vi "Graph InitScale(XY).vi"(8 "error in (no error)":errorcluster caption="エラー入力（エラーなし）", 9 "XYグラフ(Nプロット)":cluster{"X配列":dbl[], "Y配列":dbl[]}[](array[cluster]), 10 "ChName(XY)":string[](array[string]), 11 "XYグラフ(ref)":refnum<vi>) -> (0 "error out":errorcluster caption="エラー出力", 2 "OK":bool)   [LabVIEW 2014]
panel:
  in  "SAVE":bool
  in  "LOAD":bool
  in  "停止":bool
  in  "Y軸データ":T1(array[cluster])
  in  "プロットデータ":T2(array[cluster]) {"MAX" format="%#_6f"; "MIN" format="%#_6f"; "Y軸" items=["回転数", "A2", "A3", "A44", "A5", "A6", "A7", "A8"]}
  # "最大値"
  # "最小値"
  # "Y軸"
  # "表示範囲外！"
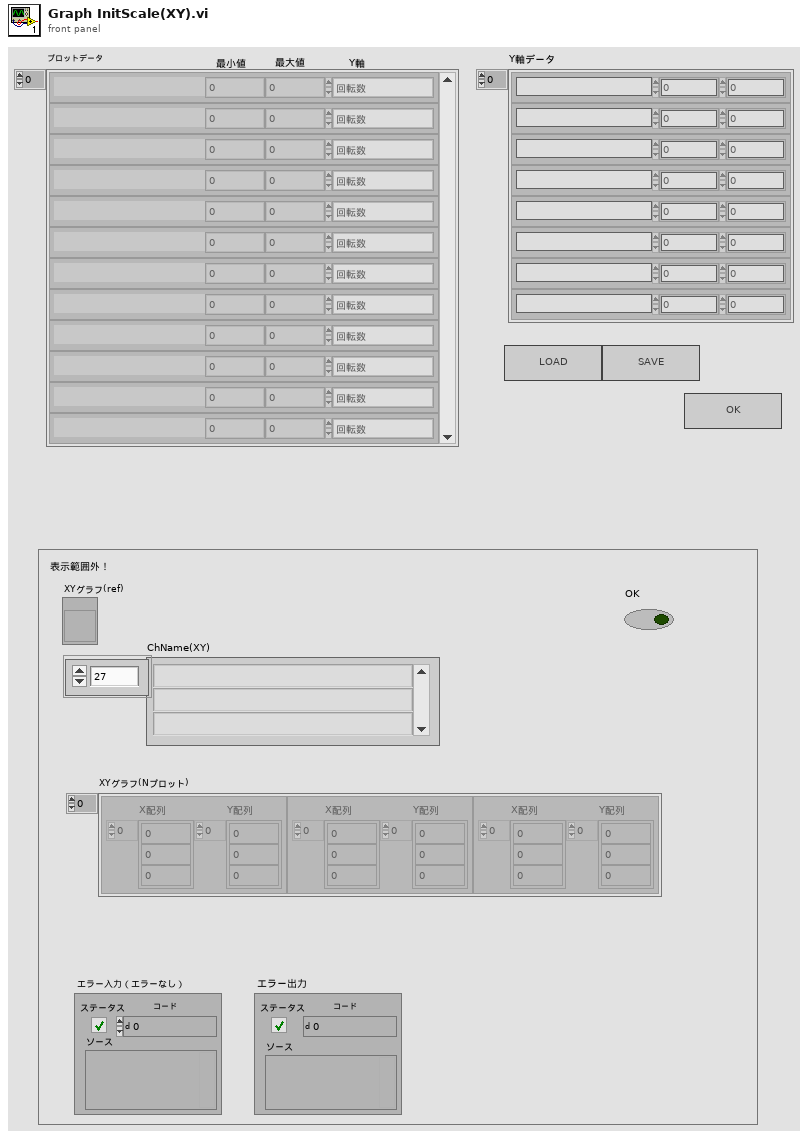
[diagram p1: front panel]
types:
  T1 = cluster{"YLegName":string, "MIN":dbl, "MAX":dbl}[]
  T2 = cluster{"CH名称":string, "MIN":dbl, "MAX":dbl, "Y軸":u16}[]
  T3 = enum32{"Invalid", "Standard", "Closed", "Hidden", "Minimized", "Maximized"}
  T4 = cluster{"CH名称":string, "MIN":dbl, "MAX":dbl, "Y軸":u16}
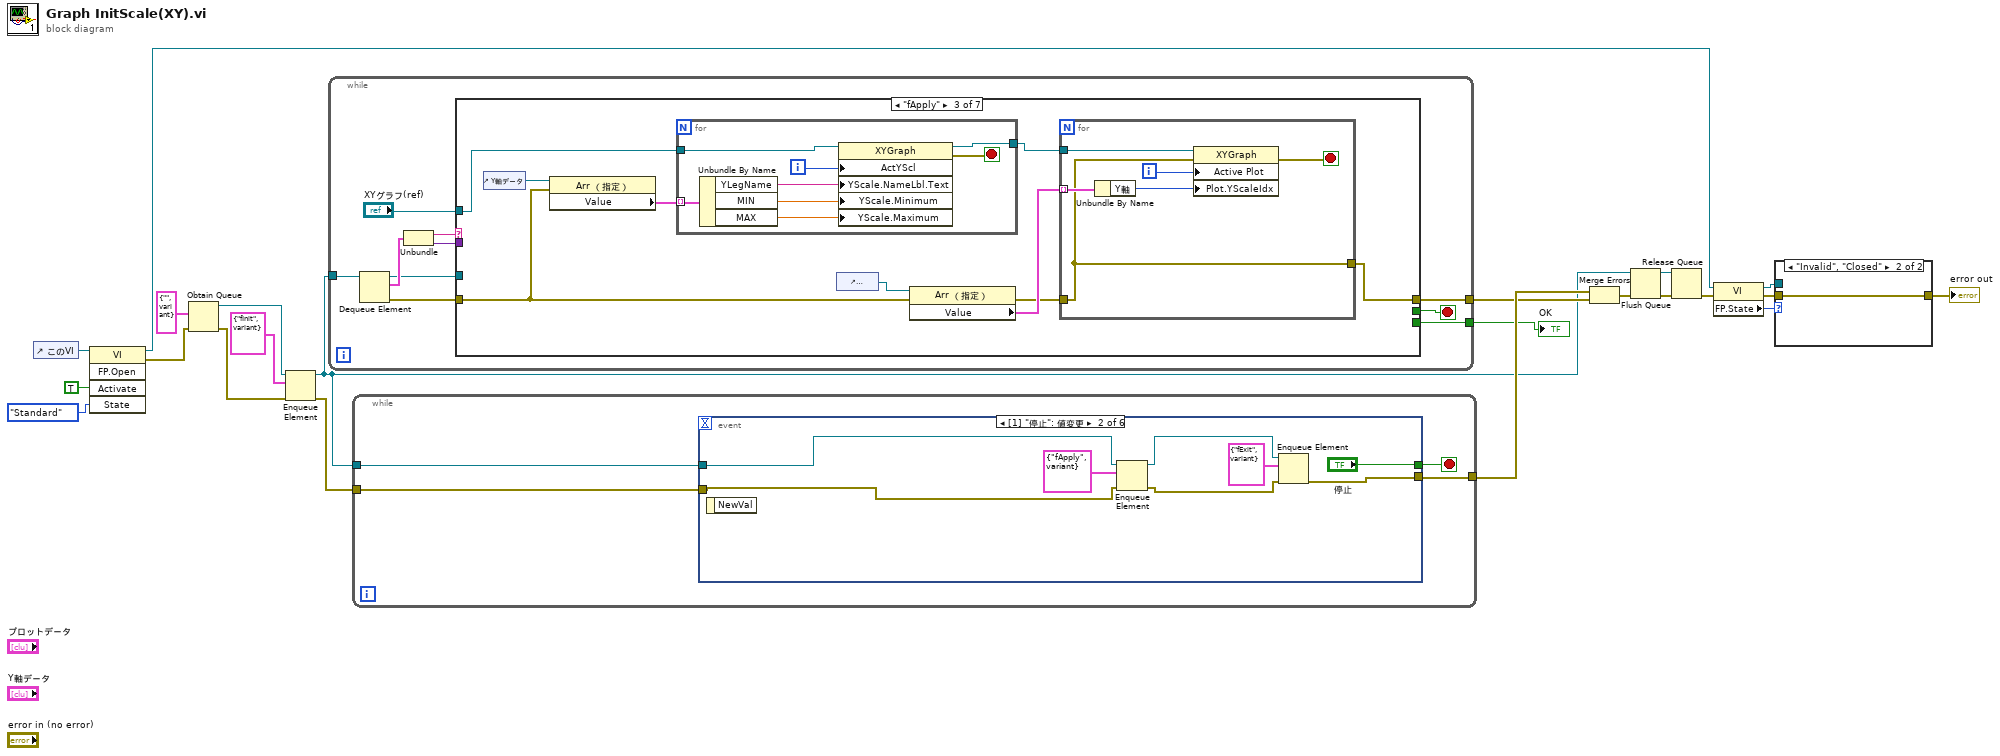
[diagram p0: block diagram]
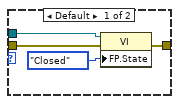
[diagram p2: hidden frame]
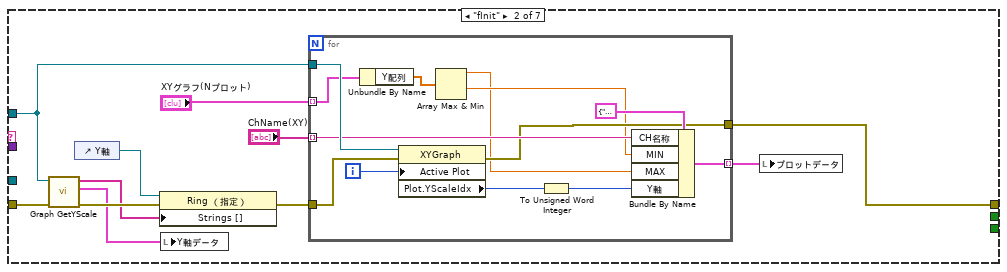
[diagram p4: hidden frame]
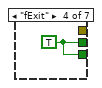
[diagram p5: hidden frame]
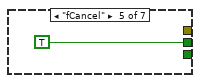
[diagram p6: hidden frame]
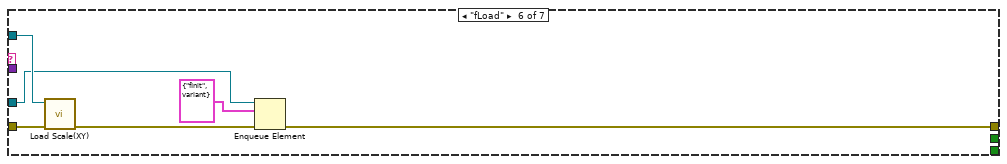
[diagram p7: hidden frame]
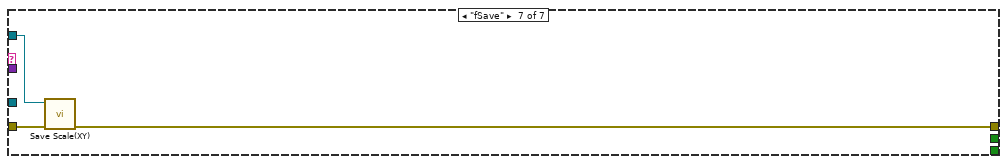
[diagram p8: hidden frame]
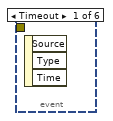
[diagram p9: hidden frame]
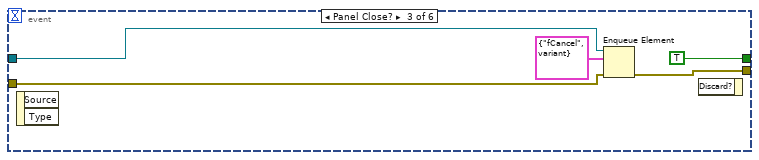
[diagram p10: hidden frame]
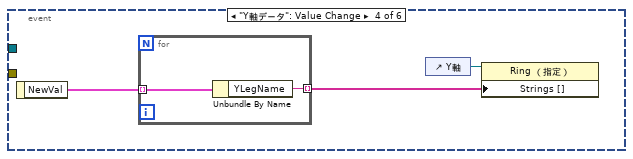
[diagram p11: hidden frame]
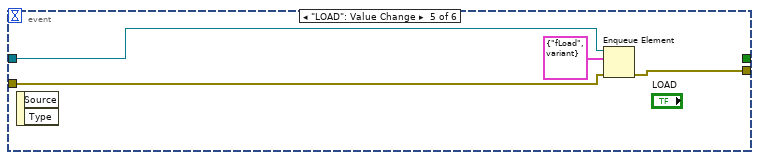
[diagram p12: hidden frame]
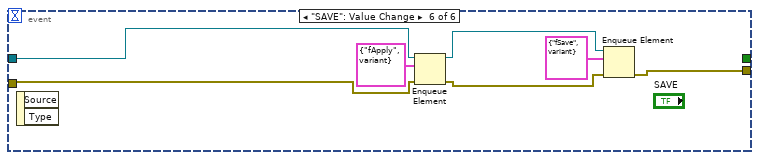
[diagram p13: hidden frame]
diagram:
  n1 = control-ref of="このVI"() -> (w17:refnum<vi>)
  n2 = invoke class="VI" method="FP.Open"(reference=w17, "Activate"=TRUE ("アクティブ化?"), "State"=T3."Standard" ("状態")) -> (reference out=w6:refnum<vi>, error out=w14:errorcluster)  [unwired: 2 in, 3 out]
  n3 = Obtain Queue(element data type=cluster{string, variant} {"", variant}, error in (no error)=w14) -> (queue out=w18:refnum<queue>, error out=w21:errorcluster)  [unwired: 3 in, 1 out]
  n4 = Enqueue Element(queue=w18, element=cluster{string, variant} {"fInit", variant} ("要素"), error in (no error)=w21) -> (queue out=w10:refnum<queue>, error out=w20:errorcluster)  [unwired: 1 in, 1 out]
  n5 = while {
    tunnel: w10 -> [w32]
    tunnel: [w27] -> w12
    tunnel: [w25] -> w7
    stop <- w28 stop-if-true
    n6 = Dequeue Element(queue=w32) -> (queue out=w24:refnum<queue>, element=w31:cluster{string, variant}, error out=w26:errorcluster)  [unwired: 2 in, 1 out]
    n7 = Unbundle(w31) -> (w30:string, w29:variant)
    n8 = case shown="\"fApply\"" w30 {
      tunnel: w29 -> [_ _ _ _ _ _ _]
      tunnel: [_ _ _ w80 TRUE _ _] -> w28
      tunnel: [_ w34 w57 _ _ w82 w88] -> w27
      tunnel: w26 -> [_ w35 w59 _ _ w86 w90]
      tunnel: "XYグラフ(ref)" -> [_ w36 w60 _ _ w87 w89]
      tunnel: [_ _ _ w80 _ _ _] -> w25
      tunnel: w24 -> [_ _ _ _ _ w84 _]
      frame "FALSE", Default {
      }
      frame "fInit" {
        n9 = call "Graph GetYScale.vi"("err in"=w35, "GraphChart入力"=w36) -> ("err out"=w42:errorcluster, "Y軸データ"=w38:T1, "Y軸名称"=w41:string[])  [unwired: 7 in]
        n10 = control-ref of="Y軸"() -> (w43:refnum<vi>)
        n11 = property class="Ring （指定）"(reference=w43, error in=w42, "Strings []"=w41) -> (error out=w40:errorcluster)  [unwired: 1 out]
        n12 = local write "Y軸データ"(w38) -> ()
        n13 = for {
          tunnel: "ChName(XY)" -> [w52] mode=indexing
          tunnel: w36 -> [w56]
          tunnel: "XYグラフ(Nプロット)" -> [w48] mode=indexing
          tunnel: w40 -> [w54]
          tunnel: [w49] -> w39 mode=indexing
          tunnel: [w46] -> w34
          i -> [w55]
          n14 = Unbundle By Name(w48) -> ("Y配列"=w47:dbl[])
          n15 = property class="XYGraph"(reference=w56, error in=w54, "Active Plot"=w55) -> (error out=w46:errorcluster, "Plot.YScaleIdx"=w51:u32)  [unwired: 1 out]
          n16 = Array Max & Min(array=w47) -> (max value=w44:dbl, min value=w45:dbl)  [unwired: 2 out]
          n17 = To Unsigned Word Integer(number=w51) -> (unsigned 16bit integer=w50:u16)
          n18 = Bundle By Name(cluster=T4 {"CH名称"="", "MIN"=0.0, "MAX"=0.0, "Y軸"=0} ("クラスタ"), "CH名称"=w52, "MIN"=w45, "MAX"=w44, "Y軸"=w50) -> (w49:T4)
        }
        n19 = local write "プロットデータ"(w39) -> ()
      }
      frame "fApply" {
        n20 = control-ref of="Y軸データ"() -> (w65:refnum<vi>)
        n21 = property class="Arr （指定）"(reference=w65, error in=w59) -> ("Value"=w64:T1)  [unwired: 2 out]
        n22 = for {
          tunnel: w60 -> [w79]
          tunnel: w64 -> [w77] mode=indexing
          tunnel: [w72] -> w61
          i -> [w78]
          stop <- w73 stop-if-true
          n23 = Unbundle By Name(w77) -> ("YLegName"=w76:string, "MIN"=w75:dbl, "MAX"=w74:dbl)
          n24 = property class="XYGraph"(reference=w79, "ActYScl"=w78, "YScale.NameLbl.Text"=w76, "YScale.Minimum"=w75, "YScale.Maximum"=w74) -> (reference out=w72:refnum<vi>, error out=w73:errorcluster)  [unwired: 1 in]
        }
        n25 = control-ref of="プロットデータ"() -> (w63:refnum<vi>)
        n26 = property class="Arr （指定）"(reference=w63, error in=w59) -> (error out=w58:errorcluster, "Value"=w62:T2)  [unwired: 1 out]
        n27 = for {
          tunnel: w62 -> [w71] mode=indexing
          tunnel: w61 -> [w70]
          tunnel: w58 -> [w66]
          tunnel: [w66] -> w57
          i -> [w69]
          stop <- w67 stop-if-true
          n28 = Unbundle By Name(w71) -> ("Y軸"=w68:u16)
          n29 = property class="XYGraph"(reference=w70, error in=w66, "Active Plot"=w69, "Plot.YScaleIdx"=w68) -> (error out=w67:errorcluster)  [unwired: 1 out]
        }
      }
      frame "fExit" {
        w80 = TRUE
      }
      frame "fCancel" {
      }
      frame "fLoad" {
        n30 = call "Load Scale(XY).vi"("err in"=w86, "XYGraph入力"=w87) -> ("err out"=w83:errorcluster)  [unwired: 9 in]
        n31 = Enqueue Element(queue=w84, element=cluster{string, variant} {"fInit", variant} ("要素"), error in (no error)=w83) -> (error out=w82:errorcluster)  [unwired: 1 in, 2 out]
      }
      frame "fSave" {
        n32 = call "Save Scale(XY).vi"("err in"=w90, "WaveformGraph入力"=w89) -> ("error out"=w88:errorcluster)  [unwired: 9 in]
      }
    }
  }
  "OK" <- w7
  n33 = while {
    tunnel: w10 -> [w93]
    tunnel: w20 -> [w92]
    tunnel: [w91] -> w13
    stop <- w94 stop-if-true
    n34 = event shown="[1] \"停止\": 値変更" {
      selector: _ -> [_ _ _ _ _ _]
      dyn-events: _ -> [_ _ _ _ _ _]
      timeout: _ -> [_ _ _ _ _ _]
      tunnel: [_ "停止" TRUE ("停止") _ _ _] -> w94
      tunnel: w93 -> [_ w98 w105 _ w115 w120]
      tunnel: w92 -> [_ w95 w104 _ w114 w117]
      tunnel: [_ w100 w103 _ w113 w122] -> w91
      event Timeout {
        n35 = event-data() -> ()  [unwired: 1 in, 3 out]
      }
      event "停止": Value Change {
        n36 = event-data() -> ()  [unwired: 1 in, 1 out]
        n37 = Enqueue Element(queue=w98, element=cluster{string, variant} {"fApply", variant} ("要素"), error in (no error)=w95) -> (queue out=w97:refnum<queue>, error out=w96:errorcluster)  [unwired: 1 in, 1 out]
        n38 = Enqueue Element(queue=w97, element=cluster{string, variant} {"fExit", variant} ("要素"), error in (no error)=w96) -> (error out=w100:errorcluster)  [unwired: 1 in, 2 out]
      }
      event Panel Close? {
        n39 = event-data() -> ()  [unwired: 1 in, 2 out]
        n40 = Enqueue Element(queue=w105, element=cluster{string, variant} {"fCancel", variant} ("要素"), error in (no error)=w104) -> (error out=w103:errorcluster)  [unwired: 1 in, 2 out]
        n41 = event-data() -> ()  [unwired: 2 in, 1 out]
      }
      event "Y軸データ": Value Change {
        n42 = event-data() -> ("NewVal"=w110:T1)  [unwired: 1 in]
        n43 = for {
          tunnel: w110 -> [w112] mode=indexing
          tunnel: [w111] -> w108 mode=indexing
          n44 = Unbundle By Name(w112) -> ("YLegName"=w111:string)
        }
        n45 = control-ref of="Y軸"() -> (w109:refnum<vi>)
        n46 = property class="Ring （指定）"(reference=w109, "Strings []"=w108) -> ()  [unwired: 1 in, 2 out]
      }
      event "LOAD": Value Change {
        n47 = event-data() -> ()  [unwired: 1 in, 2 out]
        n48 = Enqueue Element(queue=w115, element=cluster{string, variant} {"fLoad", variant} ("要素"), error in (no error)=w114) -> (error out=w113:errorcluster)  [unwired: 1 in, 2 out]
      }
      event "SAVE": Value Change {
        n49 = event-data() -> ()  [unwired: 1 in, 2 out]
        n50 = Enqueue Element(queue=w120, element=cluster{string, variant} {"fApply", variant} ("要素"), error in (no error)=w117) -> (queue out=w119:refnum<queue>, error out=w118:errorcluster)  [unwired: 1 in, 1 out]
        n51 = Enqueue Element(queue=w119, element=cluster{string, variant} {"fSave", variant} ("要素"), error in (no error)=w118) -> (error out=w122:errorcluster)  [unwired: 1 in, 2 out]
      }
    }
  }
  n52 = Merge Errors(w13, w12) -> (w11:errorcluster)
  n53 = Flush Queue(queue=w10, error in (no error)=w11) -> (queue out=w8:refnum<queue>, error out=w9:errorcluster)  [unwired: 1 out]
  n54 = Release Queue(queue=w8, error in (no error)=w9) -> (error out=w5:errorcluster)  [unwired: 1 in, 2 out]
  n55 = property class="VI"(reference=w6, error in=w5) -> (reference out=w3:refnum<vi>, error out=w2:errorcluster, "FP.State"=w4:T3)
  n56 = case shown="\"Invalid\", \"Closed\"" w4 {
    tunnel: w3 -> [w126 _]
    tunnel: w2 -> [w125 w128]
    tunnel: [w124 w128] -> w1
    frame Default {
      n57 = property class="VI"(reference=w126, error in=w125, "FP.State"=T3."Closed" ("フロントパネルウィンドウ:状態")) -> (error out=w124:errorcluster)  [unwired: 1 out]
    }
    frame "Invalid", "Closed" {
    }
  }
  "error out" <- w1
